vi "LevMar - derivative.vi"(1 "Target Function in":refnum<vi>, 2 "Coefficients":dbl[](array[numeric]) caption="A" format="%0.2f") -> (5 "Target Function out":refnum<vi>, 6 "F":dbl[](array[numeric]), 9 "dF/dA":dbl[][](array[numeric]) format="%0.5f")   [LabVIEW 2009]
panel:
  # "dérivée partielle"
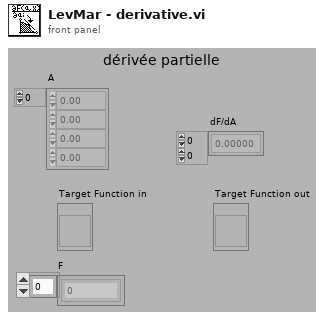
[diagram p1: front panel]
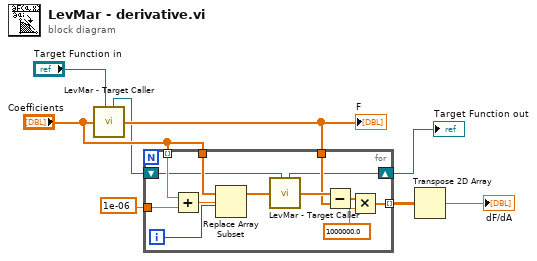
[diagram p0: block diagram]
diagram:
  n1 = call "LevMar - Target Caller.vi"("A"="Coefficients", "Target Function in"="Target Function in") -> ("Target Function out"=w1:refnum<vi>, "F"=w7:dbl[])
  "F" <- w7
  n2 = for {
    tunnel: [w19] -> w8 mode=indexing
    tunnel: "Coefficients" -> [w15] mode=indexing
    tunnel: "Coefficients" -> [w18]
    tunnel: w7 -> [w13]
    tunnel: 1e-06 -> [w12]
    shift-right: [w9] -> w3
    shift-left: w1 -> [w10]
    i -> [w16]
    n3 = Add(x=w15, y=w12) -> (x+y=w17:dbl)
    n4 = Replace Array Subset(array=w18, new element=w17, index=w16) -> (w11:dbl[])
    n5 = call "LevMar - Target Caller.vi"("A"=w11, "Target Function in"=w10) -> ("Target Function out"=w9:refnum<vi>, "F"=w14:dbl[])
    n6 = Subtract(x=w14, y=w13) -> (x-y=w20:dbl[])
    n7 = Multiply(x=w20, y=1000000.0) -> (x*y=w19:dbl[])
  }
  "Target Function out" <- w3
  n8 = Transpose 2D Array(2D array=w8) -> (transposed array=→"dF/dA":dbl[][])
